vi "CRYStrip step extension.vi"(10 "Categories":string[](array[string]), 11 "Step name w/ extension":string) -> (0 "Category number":i32, 1 "Category (full name)":string, 2 "Extension (3-letter category)":string, 3 "Step name (base)":string)   [LabVIEW 2013]
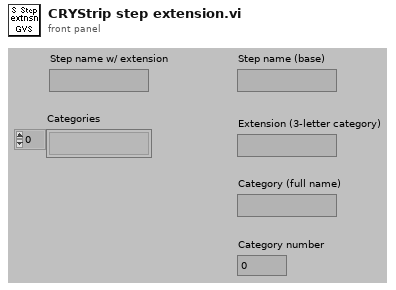
[diagram p1: front panel]
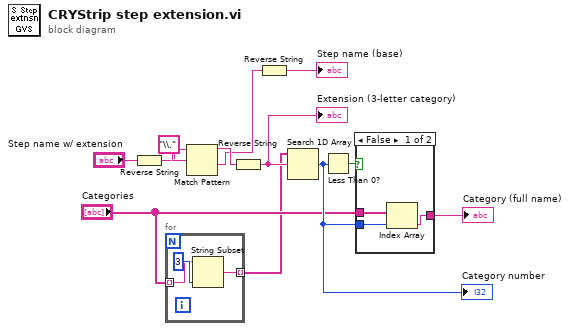
[diagram p0: block diagram]
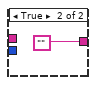
[diagram p2: hidden frame]
diagram:
  n1 = Reverse String(1:"Step name w/ extension") -> (0:w6:string)
  n2 = for {
    tunnel: "Categories" -> [w14] mode=indexing
    tunnel: [w13] -> w1 mode=indexing
    n3 = String Subset(string=w14, length (rest)=3 ("length")) -> (substring=w13:string)  [unwired: 1 out]
  }
  n4 = Match Pattern(string=w6, regular expression="\\.") -> (before substring=w5:string, after substring=w4:string)  [unwired: 3 out]
  n5 = Reverse String(1:w5) -> (0:w2:string)
  "Extension (3-letter category)" <- w2
  n6 = Reverse String(1:w4) -> (0:→"Step name (base)":string)
  n7 = Search 1D Array(1D array=w1, element=w2) -> (index of element=w10:i32)  [unwired: 1 out]
  "Category number" <- w10
  n8 = Less Than 0?(x=w10) -> (x < 0?=w11:bool)
  n9 = case shown="False" w11 {
    tunnel: "Categories" -> [w18 _]
    tunnel: w10 -> [w16 _]
    tunnel: [w17 ""] -> w9
    frame False {
      n10 = Index Array(array=w18, index=w16) -> (element=w17:string)
    }
    frame True {
    }
  }
  "Category (full name)" <- w9
